vi "Load and decimate relevant raw data.vi"(8 "error in (no error)":errorcluster) -> (0 "error out":errorcluster, 1 "Data reference":refnum<data-value>, 2 "Total # of loaded points":i32, 3 "X-axis max/min (across all loaded data types)":cluster{"X-axis max":dbl, "X-axis min":dbl}, 5 "Sorted Pointers":i32[](array[numeric]))   [LabVIEW 2013]
uses:
  xcontrol/Interface VIs/Interface typedefs/Interface-Data array.ctl
  xcontrol/Interface VIs/Interface typedefs/Interface-Data format definition.ctl
  xcontrol/Typedefs/Xctl-XY data type definition.ctl
  xcontrol/Typedefs/Xctrl-ROI type enum.ctl
  Global variables/gl_Functional Imaging-Global variables.vi
  xcontrol/XGrapher.xctl
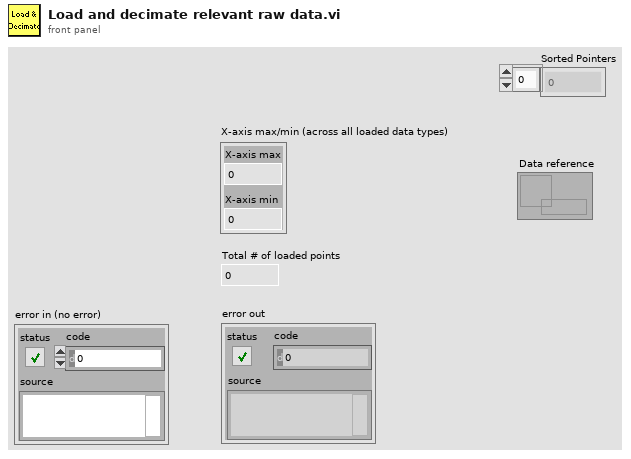
[diagram p1: front panel]
types:
  T1 = typedef "Functional Imging UI Refs.ctl" = cluster{"Menu ref":refnum<k9>, "Image control":refnum<vi>, "VI ref":refnum<vi>, "XGrapher":refnum<vi>, "Smoothing":refnum<vi>, "POI Averaging":refnum<vi>, "Normalize":refnum<vi>, "POI data points in each trial":refnum<vi>, "Channel":refnum<vi>, "Experiment data folder path":refnum<vi>, "[ROI vis]":refnum<vi>, "[Groups] visbl":T2, "Group Name":refnum<vi>, "POI index":refnum<vi>, "Trial No.":refnum<vi>, "Intensity Zoom":refnum<vi>, "Trial Cursor Enabled":refnum<vi>, "Number of Trials (ind 1)":refnum<vi>, "Number of Trials (ind 2)":refnum<vi>, "MiniScans Available":refnum<vi>, "POI Available":refnum<vi>, "Defer graph updates":refnum<vi>, "Waveform selector":refnum<vi>, "#of selected POI":refnum<vi>, "#of selected MiniScans":refnum<vi>, "#of selected groups":refnum<vi>, "Max Z-Projection":refnum<vi>, "Z-Plane Selector":refnum<vi>, "Index of miniscan point to visualise":refnum<vi>, "ROI vis. mode":refnum<vi>, "Total # of points":refnum<vi>, "Index of group clicked on":refnum<vi>, "Pane 1":refnum<vi>, "Pane 2":refnum<vi>, "Pane 3":refnum<vi>, "Pane 4":refnum<vi>, "Pane 5":refnum<vi>, "Pane 6":refnum<vi>, "Deselect all ROI":refnum<vi>, "Deselect all groups":refnum<vi>}
  T2 = typedef "Groups array referecne.ctl" = refnum<vi>
  T3 = typedef "Interface-Data array.ctl" = T4[]
  T4 = typedef "Interface-Data format definition.ctl" = cluster{"Plot.Plot Name":string, "Data":T5, "Timeline data":T5, "Type":T6, "Points per cycle":u16, "ROI number":u16}
  T5 = typedef "XGrapher.xctl/Xctl-XY data type definition.ctl" = cluster{"X-Axis values":sgl[], "Y-Axis values (s)":i32[]}
  T6 = typedef "Xctrl-ROI type enum.ctl" = enum16{"POI", "Mini-scan", "Group"}
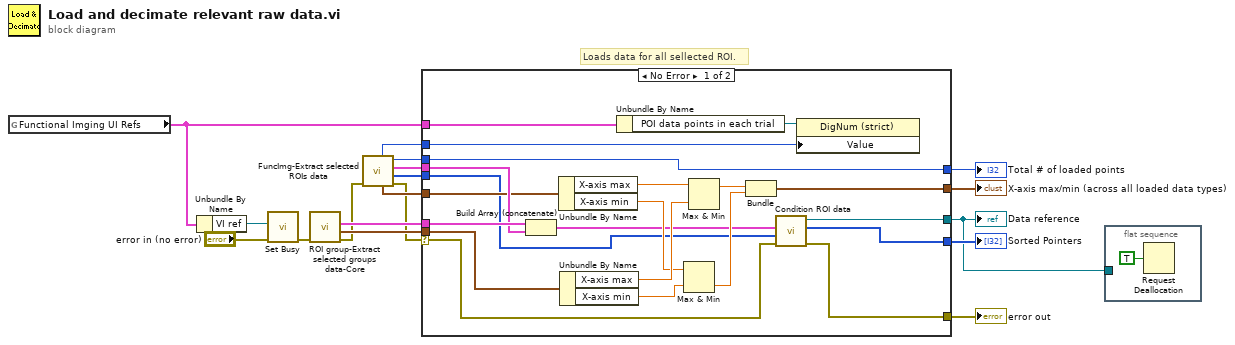
[diagram p0: block diagram]
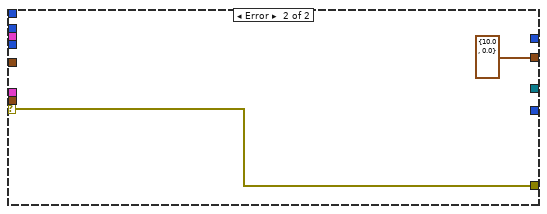
[diagram p2: hidden frame]
diagram:
  # "Loads data for all sellected ROI."
  n1 = global read "gl_Functional Imaging-Global variables.vi" "Functional Imging UI Refs"() -> (w2:T1)
  n2 = Unbundle By Name(w2) -> ("VI ref"=w1:refnum<vi>)
  n3 = call <vilib>:"Set Busy.vi"("error in (no error)"="error in (no error)", "VI reference (current VI)"=w1) -> ("error out"=w4:errorcluster)  [unwired: 8 in, 1 out]
  n4 = call "ROI group-Extract selected groups data-Core.vi"("error in"=w4) -> ("Error out"=w7:errorcluster, "X-axis max/min"=w14:cluster{"X-axis max":dbl, "X-axis min":dbl}, "Data for ticked Groups"=w15:T3)  [unwired: 8 in]
  n5 = call "FuncImg-Extract selected ROIs data.vi"("error in (no error)"=w7) -> ("error out"=w8:errorcluster, "ROI numbers"=w10:i32[], "Data for ticked ROI"=w11:T3, "Total number of points"=w12:i32, "X-axis max/min"=w9:cluster{"X-axis max":dbl, "X-axis min":dbl}, "Points in each trial"=w13:i32)  [unwired: 5 in]
  n6 = case shown="No Error" w8 {
    selector: w8 -> [w23 w41]
    tunnel: [w24 w41] -> w18
    tunnel: [w28 _] -> w17
    tunnel: [w38 cluster{dbl, dbl} {10.0, 0.0}] -> w16
    tunnel: w15 -> [w31 _]
    tunnel: w14 -> [w30 _]
    tunnel: w13 -> [w29 _]
    tunnel: w12 -> [w28 _]
    tunnel: w11 -> [w27 _]
    tunnel: w10 -> [w20 _]
    tunnel: w9 -> [w26 _]
    tunnel: [w22 _] -> w6
    tunnel: [w25 _] -> w5
    tunnel: w2 -> [w19 _]
    frame No Error {
      n7 = Build Array (concatenate)(w31, w27) -> (w21:T3)
      n8 = Unbundle By Name(w26) -> ("X-axis max"=w37:dbl, "X-axis min"=w34:dbl)
      n9 = Unbundle By Name(w30) -> ("X-axis max"=w36:dbl, "X-axis min"=w33:dbl)
      n10 = Unbundle By Name(w19) -> ("POI data points in each trial"=w39:refnum<vi>)
      n11 = Max & Min(x=w34, y=w33) -> (min(x,y)=w32:dbl)  [unwired: 1 out]
      n12 = Max & Min(x=w37, y=w36) -> (max(x,y)=w35:dbl)  [unwired: 1 out]
      n13 = Bundle(w35, w32) -> (w38:cluster{dbl, dbl})  [unwired: 1 in]
      n14 = call "Condition ROI data.vi"("error in (no error)"=w23, "ROI numbers"=w20, "Data for ticked ROI"=w21) -> ("error out"=w24:errorcluster, "Sorted Pointers"=w22:i32[], "Data reference"=w25:refnum<data-value>)  [unwired: 6 in]
      n15 = property class="DigNum (strict)"(reference=w39, "Value"=w29) -> ()  [unwired: 1 in, 2 out]
    }
    frame Error {
    }
  }
  "error out" <- w18
  "Total # of loaded points" <- w17
  "X-axis max/min (across all loaded data types)" <- w16
  "Sorted Pointers" <- w6
  "Data reference" <- w5
  n16 = flat-sequence {
    tunnel: w5 -> [_]
    frame #0 {
      n17 = Request Deallocation(TRUE ("flag")) -> ()
    }
  }
